vi "RF_calibration_33220Ascan.vi"() -> ()   [LabVIEW 2020]
uses:
  instr.lib/Tektronix TDS 200 1000 2000 Series/Tektronix TDS 200 1000 2000 Series.lvlib
  ion_trap_control_vi-master/instr.lib/Agilent 33XXX Series/Agilent 33XXX Series.lvlib
panel:
  out "Graph 3":cluster{dbl[], dbl[]}(graph)={[200.0, 300.0, 300.0, 300.0, 300.0], [0.0544000007, 0.0544000007, 0.0903999954, 0.0903999954, 0.1011999995]}
  in  "COMMENT":string="TEST"
  out "Graph 2":cluster{dbl[], dbl[]}(graph)={[200.0, 300.0, 300.0, 300.0, 300.0], [1200.0, 1200.0, 2000.0, 2000.0, 2400.0]}
  out "Graph":cluster{dbl[], dbl[]}(graph)={[200.0, 300.0, 300.0, 300.0, 300.0], [160000.0, 160000.0, 160000.0, 160000.0, 160000.0]}
  in  "Tab Control":enum32{"CONFIG", "MAIN", "DIAGNOSIS"}(tab)
  in  "Agilent 33220A":refnum<visa-resource-name>="USB0::0x0D4A::0x000E::9260521::INSTR"
  in  "Columns":string[](array[string])=["SF1/SF2", "l (mm)", "FG freq (Hz)", "FG V (mVpp)", "CH1 Monitor (Vpp)", "CH2 VR (Vpp)", "CH2 Antenna (Vpp)"]
  in  "File path":path=path "C:/LabVIEW/DATA/J-PARC_202206/RF_zscans"
  in  "Tektronix":refnum<visa-resource-name>="USB0::0x0699::0x0365::C035183::INSTR"
  out "File ref (calibration)":refnum<file>
  out "Error Out":errorcluster={"status"=FALSE, "code"=1073676290, "source"="NF WF1973_74 Initialize.vi->RF_calibration_NF_WF1974_scan.vi内のVISAイベント有効"}
  in  "Measure":bool
  in  "Vamp lower lim":dbl=0.4 format="%_4f"
  in  "Vamp upper lim":dbl=3000.0 format="%_4f"
  in  "FG reset":bool
  in  "Amplitude (mVpp)":dbl=1200.0 format="%_6f"
  in  "FG Output":bool
  in  "Frequency (Hz)":dbl=160000.0 format="%_8e"
  out "Measurement index":i32
  out "CH 1 measurement":dbl=0.1011999995 format="%_6g"
  out "CH 2 measurement":dbl=3.4600000381 format="%_6g"
  out "CH3 measurement":dbl=0.00208
  in  "L (mm)":dbl=300.0
  in  "SF1 or2?":u32=1
  out "Latest measurements":dbl[][](array[numeric]) format="%_4e"
  out "index":i32[](array[numeric])
  out "error out (Agilent)":errorcluster
  out "error out (Tektronix)":errorcluster
  out "error out (file operation)":errorcluster
  in  "STOP":bool
  # "Z SCAN OF THE RF FIELD"
  # "SCAN INPUTS"
  # "FG CONTROL"
  # "TEKTRONIX READOUT"
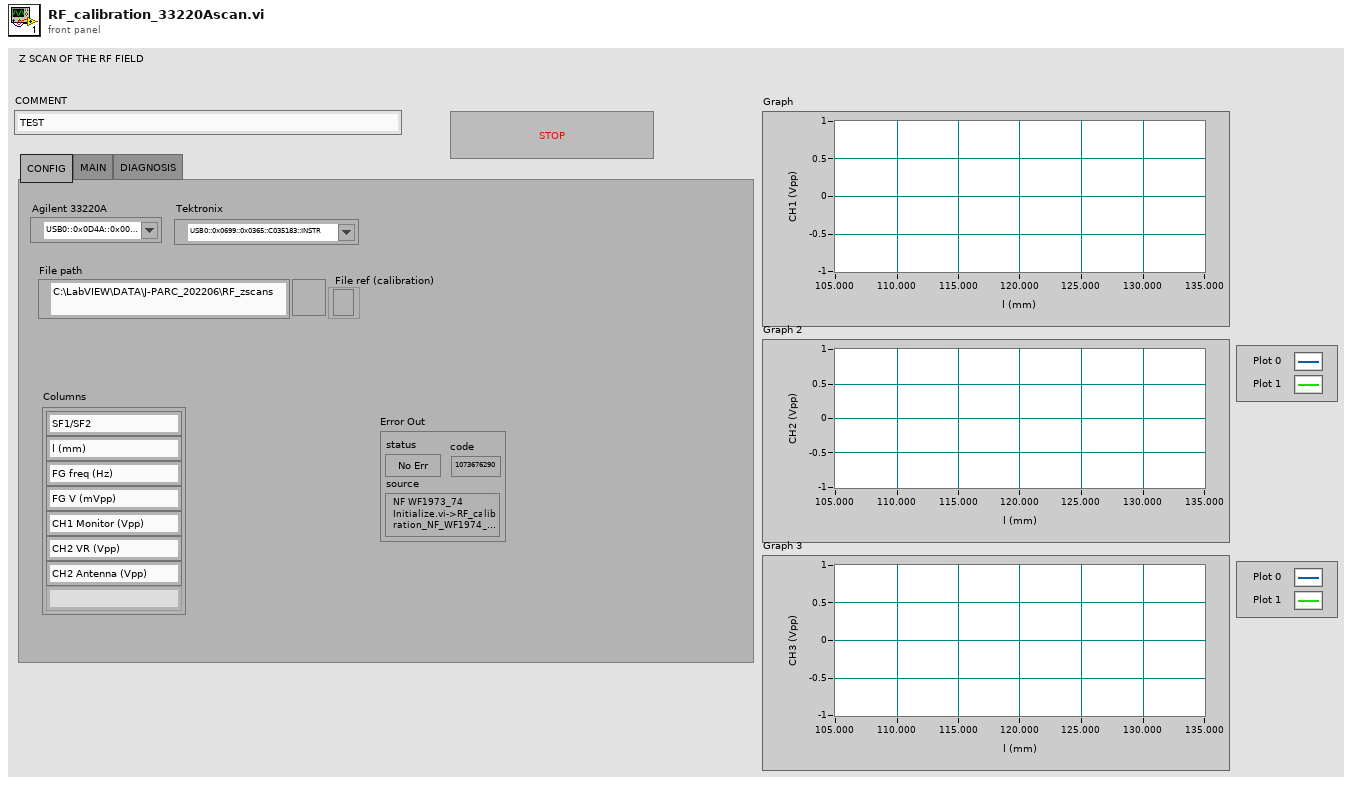
[diagram p1: front panel]
types:
  T1 = cluster{"Baud Rate":u32, "Parity":u16, "Stop Bits":u16, "Flow Control":u16}
  T2 = enum16{"open", "replace", "create", "open or create", "replace or create", "replace or create with confirmation"}
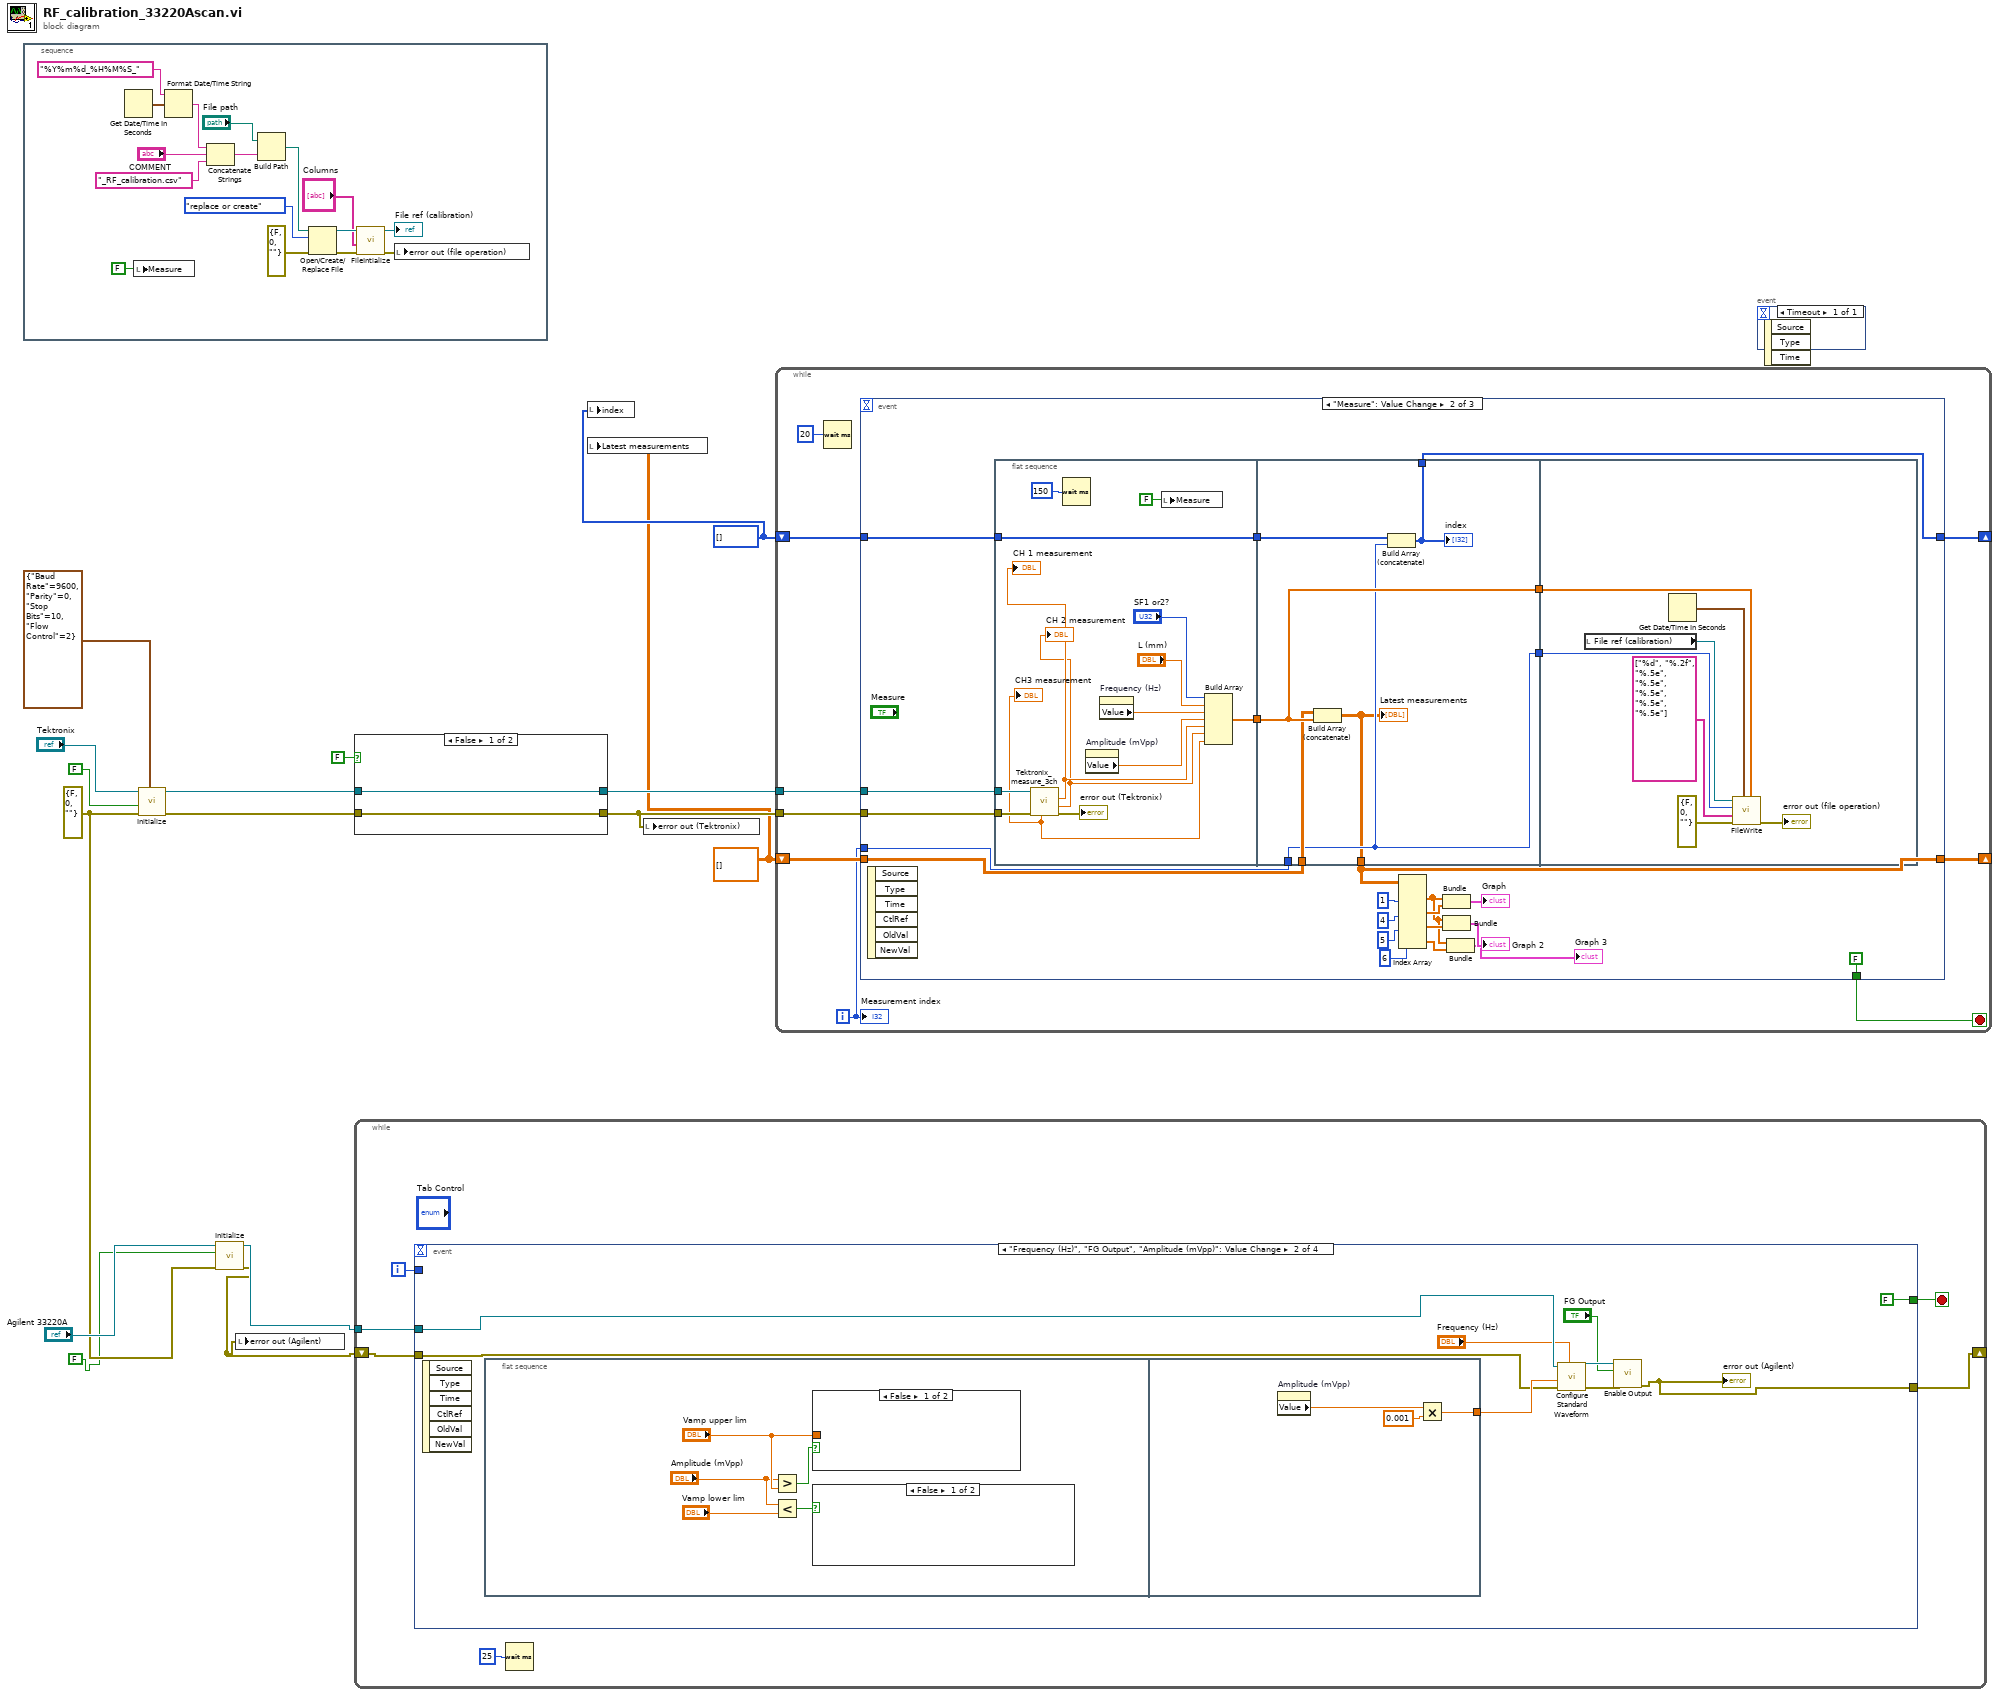
[diagram p0: block diagram]
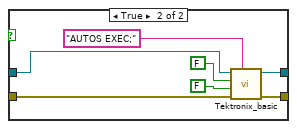
[diagram p2: hidden frame]
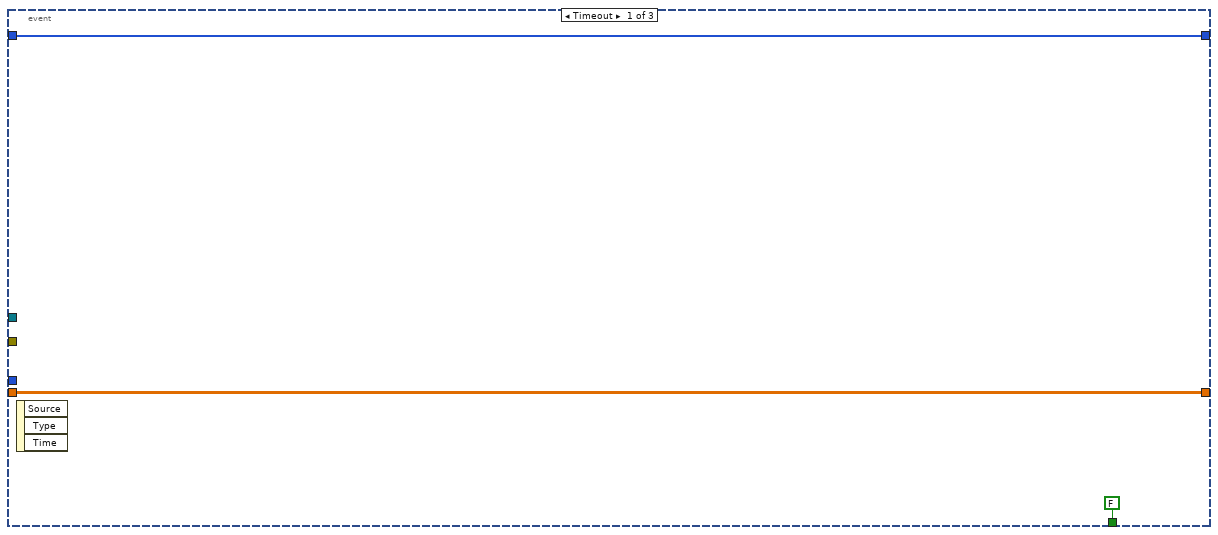
[diagram p3: hidden frame]
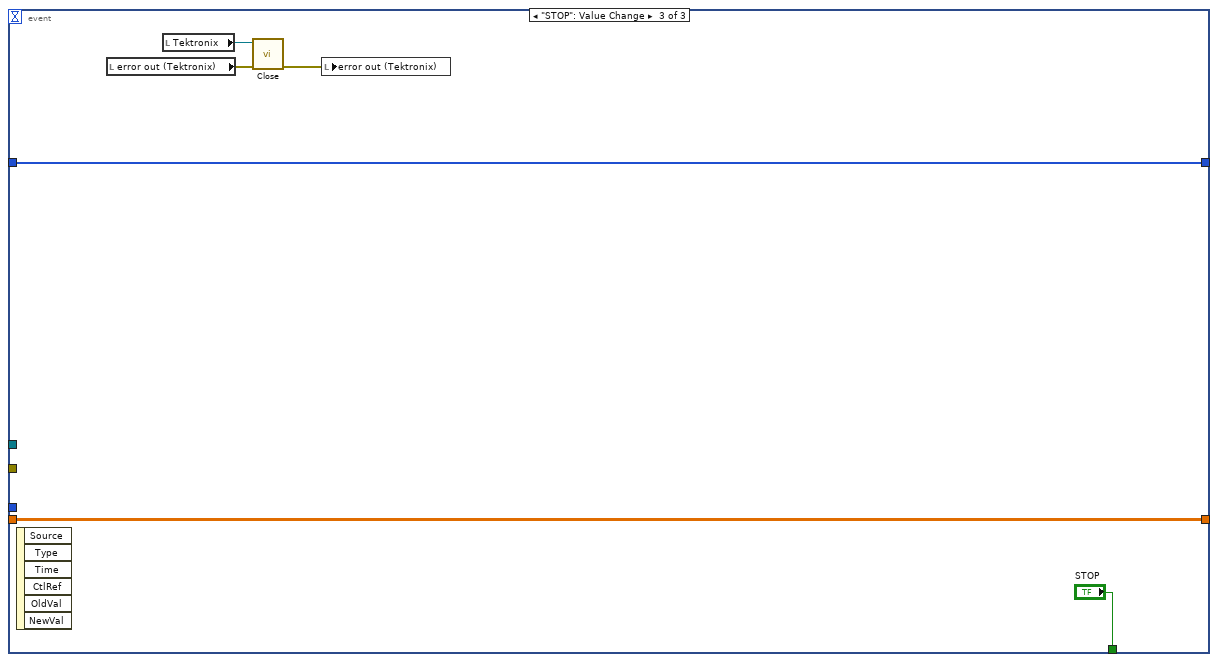
[diagram p4: hidden frame]
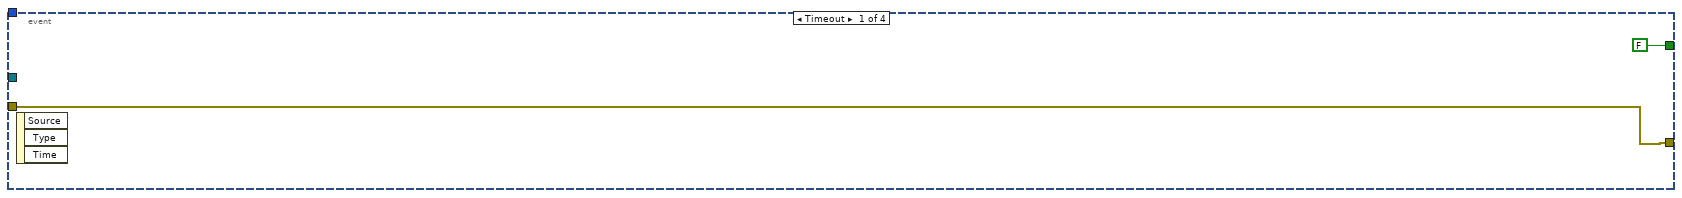
[diagram p5: hidden frame]
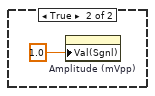
[diagram p6: hidden frame]
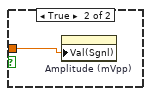
[diagram p7: hidden frame]
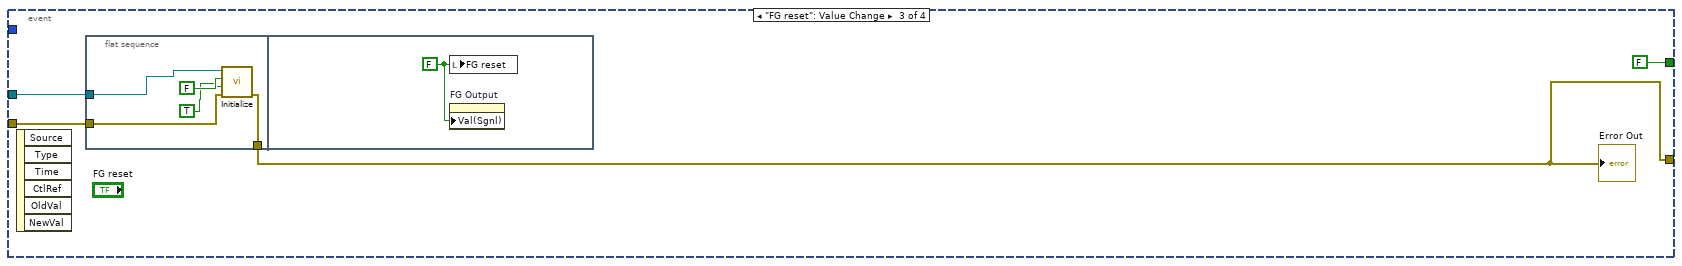
[diagram p8: hidden frame]
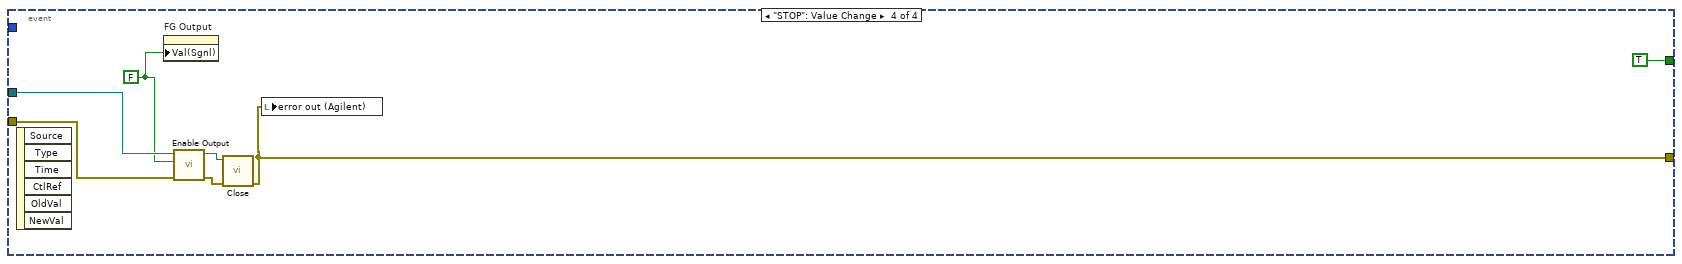
[diagram p9: hidden frame]
diagram:
  w6 = dbl[][] []
  w7 = i32[] []
  w4 = errorcluster {"status"=FALSE, "code"=0, "source"=""} ("error in (no error)")
  n1 = stacked-sequence {
    frame #0 {
      n2 = Get Date/Time In Seconds() -> (seconds since 1Jan1904=w20:timestamp)
      n3 = local write "Measure"(FALSE ("Measure")) -> ()
      n4 = Format Date/Time String(time format string (%c)="%Y%m%d_%H%M%S_", seconds (now)=w20) -> (date/time string=w18:string)  [unwired: 1 in]
      n5 = Concatenate Strings(w18, "COMMENT", "_RF_calibration.csv") -> (w31:string)
      n6 = Build Path(base path="File path", name or relative path=w31) -> (appended path=w30:path)
      n7 = Open/Create/Replace File(file path (use dialog)=w30, error in=errorcluster {"status"=FALSE, "code"=0, "source"=""}, operation (0:open)=T2."replace or create") -> (refnum out=w27:refnum<file>, error out=w28:errorcluster)  [unwired: 3 in, 1 out]
      n8 = call "FileIntialize.vi"("Error In"=w28, "Labels"="Columns", "refnum in"=w27) -> ("Error Out"=w17:errorcluster, "File Refnum"=→"File ref (calibration)":refnum<file>)  [unwired: 7 in]
      n9 = local write "error out (file operation)"(w17) -> ()
    }
  }
  n10 = call "Initialize.vi"("Serial Configuration"=T1 {"Baud Rate"=9600, "Parity"=0, "Stop Bits"=10, "Flow Control"=2}, "error in (no error)"=w4, "Reset? (T: Yes)"=FALSE, "VISA resource name"="Tektronix") -> ("error out"=w12:errorcluster, "VISA resource name out"=w11:refnum<visa-resource-name>)  [unwired: 1 in, 5 out]
  n11 = call "Initialize.vi"("error in (no error)"=w4, "ID Query (True)"=FALSE ("Reset (True)"), "VISA resource name"="Agilent 33220A") -> ("error out"=w1:errorcluster, "VISA resource name out"=w2:refnum<visa-resource-name>)  [unwired: 7 in]
  n12 = local write "error out (Agilent)"(w1) -> ()
  n13 = case shown="False" FALSE {
    tunnel: w12 -> [w32 w40]
    tunnel: w11 -> [w33 w39]
    tunnel: [w33 w38] -> w10
    tunnel: [w32 w37] -> w9
    frame False {
    }
    frame True {
      n14 = call "Tektronix_basic.vi"("write buffer"="AUTOS EXEC;", "error in (no error)"=w40, "Query?"=FALSE, "Error query?"=FALSE, "VISA resource name"=w39) -> ("error out"=w37:errorcluster, "VISA resource name out"=w38:refnum<visa-resource-name>)  [unwired: 4 in, 1 out]
    }
  }
  n15 = while {
    tunnel: w2 -> [w46]
    shift-right: [w41] -> _
    shift-left: w1 -> [w42]
    i -> [w43]
    stop <- w44 stop-if-true
    n16 = event shown="[1] \"Frequency (Hz)\", \"FG Output\", \"Amplitude (mVpp)\": Value Change" {
      selector: _ -> [_ _ _ _]
      dyn-events: _ -> [_ _ _ _]
      timeout: _ -> [_ _ _ _]
      tunnel: w46 -> [_ w56 w70 w83]
      tunnel: [FALSE FALSE FALSE TRUE] -> w44
      tunnel: w43 -> [_ _ _ _]
      tunnel: w42 -> [w47 w50 w69 w78]
      tunnel: [w47 w51 w68 w79] -> w41
      event Timeout {
        n17 = event-data() -> ()  [unwired: 1 in, 3 out]
      }
      event "Frequency (Hz)", "FG Output", "Amplitude (mVpp)": Value Change {
        n18 = event-data() -> ()  [unwired: 1 in, 6 out]
        n19 = flat-sequence {
          tunnel: [w66] -> w55
          frame #0 {
            n20 = Greater?(x="Amplitude (mVpp)", y="Vamp upper lim") -> (0:w61:bool)
            n21 = Less?(x="Amplitude (mVpp)", y="Vamp lower lim") -> (x < y?=w58:bool)
            n22 = case shown="False" w61 {
              tunnel: "Vamp upper lim" -> [_ w64]
              frame False {
              }
              frame True {
                n23 = property on="Amplitude (mVpp)" class="DigNum (strict)"("Val(Sgnl)"=w64) -> ()  [unwired: 2 in, 2 out]
              }
            }
            n24 = case shown="False" w58 {
              frame False {
              }
              frame True {
                n25 = property on="Amplitude (mVpp)" class="DigNum (strict)"("Val(Sgnl)"=1.0 ("Value (Signaling)")) -> ()  [unwired: 2 in, 2 out]
              }
            }
          }
          frame #1 {
            n26 = property on="Amplitude (mVpp)" class="DigNum (strict)"() -> ("Value"=w65:dbl)  [unwired: 2 in, 2 out]
            n27 = Multiply(x=w65, y=0.001) -> (x*y=w66:dbl)
          }
        }
        n28 = call "Configure Standard Waveform.vi"("Frequency (1000 Hz)"="Frequency (Hz)", "error in (no error)"=w50, "Amplitude (1)"=w55, "VISA resource name"=w56) -> ("error out"=w52:errorcluster, "VISA resource name out"=w53:refnum<visa-resource-name>)  [unwired: 6 in]
        n29 = call "Enable Output.vi"("error in (no error)"=w52, "Enable Output  (T: Enable)"="FG Output", "VISA resource name"=w53) -> ("error out"=w51:errorcluster)  [unwired: 7 in, 1 out]
        "error out (Agilent)" <- w51
      }
      event "FG reset": Value Change {
        n30 = event-data() -> ()  [unwired: 1 in, 6 out]
        n31 = flat-sequence {
          tunnel: w70 -> [w76]
          tunnel: w69 -> [w73]
          tunnel: [w72] -> w68
          frame #0 {
            n32 = call "Initialize.vi"("error in (no error)"=w73, "Reset (True)"=TRUE ("Reset(T)"), "ID Query (True)"=FALSE, "VISA resource name"=w76) -> ("error out"=w72:errorcluster)  [unwired: 6 in, 1 out]
          }
          frame #1 {
            w77 = FALSE ("Value (Signaling)")
            n33 = local write "FG reset"(w77) -> ()
            n34 = property on="FG Output" class="Bool (strict)"("Val(Sgnl)"=w77) -> ()  [unwired: 2 in, 2 out]
          }
        }
        "Error Out" <- w68
      }
      event "STOP": Value Change {
        w82 = FALSE ("Enable Output  (T: Enable)")
        n35 = event-data() -> ()  [unwired: 1 in, 6 out]
        n36 = property on="FG Output" class="Bool (strict)"("Val(Sgnl)"=w82) -> ()  [unwired: 2 in, 2 out]
        n37 = call "Enable Output.vi"("error in (no error)"=w78, "Enable Output  (T: Enable)"=w82, "VISA resource name"=w83) -> ("error out"=w80:errorcluster, "VISA resource name out"=w81:refnum<visa-resource-name>)  [unwired: 7 in]
        n38 = call "Close.vi"("error in (no error)"=w80, "VISA resource name"=w81) -> ("error out"=w79:errorcluster)  [unwired: 9 in]
        n39 = local write "error out (Agilent)"(w79) -> ()
      }
    }
    n40 = Wait (ms)(milliseconds to wait=u32 25) -> ()  [unwired: 1 out]
  }
  n41 = local write "index"(w7) -> ()
  n42 = local write "Latest measurements"(w6) -> ()
  n43 = local write "error out (Tektronix)"(w9) -> ()
  n44 = while {
    tunnel: w9 -> [w93]
    tunnel: w10 -> [w92]
    shift-right: [w91] -> _
    shift-left: w7 -> [w90]
    shift-right: [w89] -> _
    shift-left: w6 -> [w88]
    i -> [w87]
    stop <- w85 stop-if-true
    n45 = Wait (ms)(milliseconds to wait=u32 20) -> ()  [unwired: 1 out]
    n46 = event shown="[1] \"Measure\": Value Change" {
      selector: _ -> [_ _ _]
      dyn-events: _ -> [_ _ _]
      timeout: _ -> [_ _ _]
      tunnel: w93 -> [_ w118 _]
      tunnel: w92 -> [_ w117 _]
      tunnel: [w96 w113 w149] -> w91
      tunnel: w90 -> [w96 w119 w149]
      tunnel: [w95 w114 w148] -> w89
      tunnel: w88 -> [w95 w115 w148]
      tunnel: w87 -> [_ w116 _]
      tunnel: [FALSE ("STOP") FALSE ("STOP") "STOP"] -> w85
      event Timeout {
        n47 = event-data() -> ()  [unwired: 1 in, 3 out]
      }
      event "Measure": Value Change {
        n48 = event-data() -> ()  [unwired: 1 in, 6 out]
        n49 = flat-sequence {
          tunnel: [w133] -> w112
          tunnel: w119 -> [w133]
          tunnel: w118 -> [w127]
          tunnel: w117 -> [w126]
          tunnel: [w125] -> w111
          tunnel: w112 -> [w138]
          tunnel: [w139] -> w110
          tunnel: w111 -> [w139]
          tunnel: w116 -> [w136]
          tunnel: w115 -> [w137]
          tunnel: [w134] -> w114
          tunnel: [w136] -> w109
          tunnel: [w135] -> w113
          tunnel: w110 -> [w141]
          tunnel: w109 -> [w140]
          frame #0 {
            n50 = call "Tektronix_measure_3ch.vi"("error in (no error)"=w127, "VISA resource name"=w126) -> ("error out"=→"error out (Tektronix)":errorcluster, "Measurement 2"=w121:dbl, "Measurement 1"=w122:dbl, "Measurement 3"=w120:dbl)  [unwired: 2 in, 4 out]
            "CH 1 measurement" <- w122
            "CH 2 measurement" <- w121
            "CH3 measurement" <- w120
            n51 = Wait (ms)(milliseconds to wait=u32 150) -> ()  [unwired: 1 out]
            n52 = property on="Amplitude (mVpp)" class="DigNum (strict)"() -> ("Value"=w129:dbl)  [unwired: 2 in, 2 out]
            n53 = property on="Frequency (Hz)" class="DigNum (strict)"() -> ("Value"=w128:dbl)  [unwired: 2 in, 2 out]
            n54 = local write "Measure"(FALSE ("Measure")) -> ()
            n55 = Build Array("SF1 or2?", "L (mm)", w128, w129, w122, w121, w120) -> (w125:dbl[])
          }
          frame #1 {
            n56 = Build Array (concatenate)(w137, w139) -> (w134:dbl[][])
            "Latest measurements" <- w134
            n57 = Build Array (concatenate)(w138, w136) -> (w135:i32[])
            "index" <- w135
          }
          frame #2 {
            n58 = local read "File ref (calibration)"() -> (w146:refnum<file>)
            n59 = Get Date/Time In Seconds() -> (seconds since 1Jan1904=w143:timestamp)
            n60 = call "FileWrite.vi"("DataArray"=w141, "Time Stamp"=w143, "Error In"=errorcluster {"status"=FALSE, "code"=0, "source"=""}, "FileFormat"=string[] ["%d", "%.2f", "%.5e", "%.5e", "%.5e", "%.5e", "%.5e"], "Index"=w140, "refnum in"=w146) -> ("Error Out"=→"error out (file operation)":errorcluster)  [unwired: 4 in, 1 out]
          }
        }
        n61 = Index Array(array=w114, index (col) #1=1 ("無効な指標 （列）"), index (col) #2=4 ("disabled index (col)"), index (col) #3=5 ("index (row)"), index (col) #4=6 ("指標 （列）")) -> (element #1=w100:dbl[], element #2=w105:dbl[], element #3=w103:dbl[], element #4=w99:dbl[])  [unwired: 4 in]
        n62 = Bundle(w100, w105) -> (→"Graph":cluster{dbl[], dbl[]})  [unwired: 1 in]
        n63 = Bundle(w100, w103) -> (→"Graph 2":cluster{dbl[], dbl[]})  [unwired: 1 in]
        n64 = Bundle(w100, w99) -> (→"Graph 3":cluster{dbl[], dbl[]})  [unwired: 1 in]
      }
      event "STOP": Value Change {
        n65 = event-data() -> ()  [unwired: 1 in, 6 out]
        n66 = local read "error out (Tektronix)"() -> (w151:errorcluster)
        n67 = local read "Tektronix"() -> (w150:refnum<visa-resource-name>)
        n68 = call "Close.vi"("error in (no error)"=w151, "VISA resource name"=w150) -> ("error out"=w152:errorcluster)  [unwired: 9 out]
        n69 = local write "error out (Tektronix)"(w152) -> ()
      }
    }
    "Measurement index" <- w87
  }
  n70 = event shown="[0] Timeout" {
    selector: _ -> [_]
    dyn-events: _ -> [_]
    timeout: _ -> [_]
    event Timeout {
      n71 = event-data() -> ()  [unwired: 1 in, 3 out]
    }
  }
